vi "Initialize Lockin.vi"(8 "error in (no error)":errorcluster, 11 "Hardware Parameters":T1={"Scan Calibration [G/V]"=0.0, "Modulation Calibration [G/V]"=0.0, "Modulation Phase [deg]"=0.0, "Modulation Frequency [Hz]"=0.0, "Attenuation [dB]"=0, "Input Channel Count"=0, "Time constant"=7, "Sensitivity"=17, "Frequency Output Voltage [V]"=0.0, "Phase Output Voltage [V]"=0.0, "Lock-in Offset Compensation"=FALSE, "RF [GHz]"=0.0, "Q Start"=0.0, "Q End"=0.0, "Balance"=0.0, "Phase Error"=0.0, "AFC Error"=0.0, "AFC"=FALSE, "Magnet Rotation"=FALSE, "Balance Scaling Factor"=1.0, "Phase Error Scaling Factor"=1.0, "AFC Error Scaling Factor"=1.0, "Frequency Counter ID"="", "Sweep Waveform"=enum."Sawtooth", "Q-Factor Scale"=0.0, " Q-Data Scale"=0.0, " Q-Data Offset"=0.0, "Magnet Rotation Slope"=0.0, "Magnet Rotation Offset"=0.0, "Phase Sweep Resolution"=0.0, "Hardware Version Number"="", "Spectrometer ID Number"=0, "Spectrometer Name"="", "Lock in Saturation"=0.0, "Balance Threshold"=0.0, "Phase Error Threshold"=0.0, "AFC Error Threshold"=0.0, "Linear Actuator Length"=0.0, "Lock-in OK?"=FALSE, "Ignore Lock-in Comm. Failure"=FALSE, "Gradient Addresses"=[], "Gradient Calibrations [G/A*mm]"=[], "Gradient Power Supplies"=[], "Lock-in Address"="", "Magnet Type"=enum."RRI", "Camera Names"=[], "Sweep Limit [Gauss]"=0.0, "Modulation Limit [Gauss]"=0.0, "Balance Threshold Exceeded?"=FALSE, "Phase Threshold Exceeded?"=FALSE, "AFC Threshold Exceeded?"=FALSE, "Consecutive Re-tune attempts"=0, "Reverse Sweep Slope [sec]"=0.0, "Reverse Sweep Offset [G]"=0.0, "AFC Field Correction [V/MHz]"=0.0, "Active Gradients (X Y Z)"=[], "SpO2 Calibration [SpO2/V]"=1.0, "Heart Rate Calibration [BPM/V]"=1.0, "Thermocouple Channel"=""} {"Sensitivity" items=["", "2 nV", "5 nV", "10 nV", "20 nV", "50 nV", "100 nV", "200 nV", "500 nV", "1 uV", "2 uV", "5 uV", "10 uV", "20 uV", "50 uV", "100 uV", "200 uV", "500 uV", "1 mV", "2 mV", "5 mV", "10 mV", "20 mV", "50 mV", "100 mV", "200 mV", "500 mV", "1 V"]; "Time constant" items=["10 us", "20 us", "40 us", "80 us", "160 us", "320 us", "640 us", "5 ms", "10 ms", "20 ms", "50 ms", "100 ms", "200 ms", "500 ms", "1 s", "2 s", "5 s", "10 s", "20 s", "50 s", "100 s", "200 s", "500 s", "1 ks", "2 ks", "5 ks", "10 ks", "20 ks", "50 ks", "100 ks"]}) -> (0 "error out":errorcluster)   [LabVIEW 2016]
uses:
  Types/Hardware Parameters.ctl
panel:
  # "Bridge I/O"
  # "Magnet Rotation"
  # "Field Calibration"
  # "Lock In Amplifier"
  # "Spectrometer Information"
  # "DAQ Settings"
  # "Gradient Coils and Field"
  # "X"
  # "Y"
  # "Z"
  # "Q-Measurements"
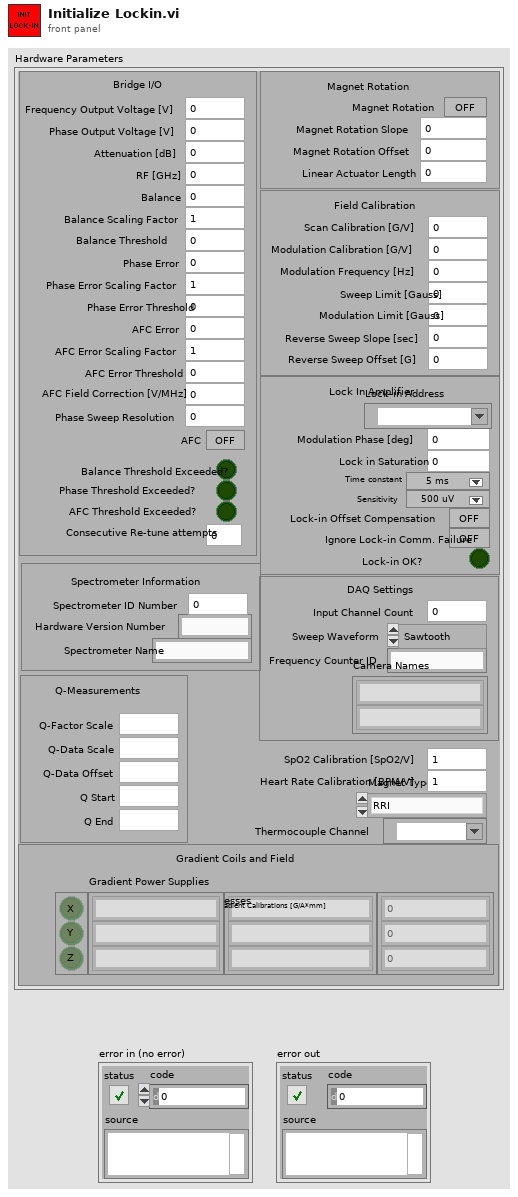
[diagram p1: front panel]
types:
  T1 = typedef "Hardware Parameters.ctl" = cluster{"Scan Calibration [G/V]":dbl, "Modulation Calibration [G/V]":dbl, "Modulation Phase [deg]":dbl, "Modulation Frequency [Hz]":dbl, "Attenuation [dB]":u16, "Input Channel Count":i32, "Time constant":u16, "Sensitivity":u16, "Frequency Output Voltage [V]":dbl, "Phase Output Voltage [V]":dbl, "Lock-in Offset Compensation":bool, "RF [GHz]":dbl, "Q Start":dbl, "Q End":dbl, "Balance":dbl, "Phase Error":dbl, "AFC Error":dbl, "AFC":bool, "Magnet Rotation":bool, "Balance Scaling Factor":dbl, "Phase Error Scaling Factor":dbl, "AFC Error Scaling Factor":dbl, "Frequency Counter ID":string, "Sweep Waveform":enum16{"Sine Wave", "Square Wave", "Sawtooth", "Triangle Wave"}, "Q-Factor Scale":dbl, " Q-Data Scale":dbl, " Q-Data Offset":dbl, "Magnet Rotation Slope":dbl, "Magnet Rotation Offset":dbl, "Phase Sweep Resolution":dbl, "Hardware Version Number":string, "Spectrometer ID Number":i32, "Spectrometer Name":string, "Lock in Saturation":dbl, "Balance Threshold":dbl, "Phase Error Threshold":dbl, "AFC Error Threshold":dbl, "Linear Actuator Length":dbl, "Lock-in OK?":bool, "Ignore Lock-in Comm. Failure":bool, "Gradient Addresses":string[], "Gradient Calibrations [G/A*mm]":dbl[], "Gradient Power Supplies":string[], "Lock-in Address":refnum<visa-resource-name>, "Magnet Type":enum16{"RRI", "BARDA", "Whole Body Permanent", "RRI Electromagnet"}, "Camera Names":string[], "Sweep Limit [Gauss]":dbl, "Modulation Limit [Gauss]":dbl, "Balance Threshold Exceeded?":bool, "Phase Threshold Exceeded?":bool, "AFC Threshold Exceeded?":bool, "Consecutive Re-tune attempts":i32, "Reverse Sweep Slope [sec]":dbl, "Reverse Sweep Offset [G]":dbl, "AFC Field Correction [V/MHz]":dbl, "Active Gradients (X Y Z)":bool[], "SpO2 Calibration [SpO2/V]":dbl, "Heart Rate Calibration [BPM/V]":dbl, "Thermocouple Channel":tag}
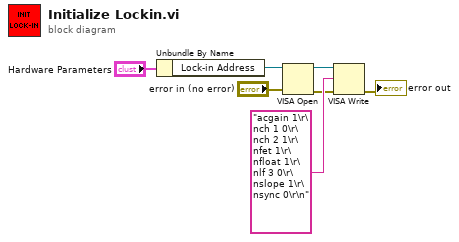
[diagram p0: block diagram]
diagram:
  n1 = Unbundle By Name("Hardware Parameters") -> ("Lock-in Address"=w1:refnum<visa-resource-name>)
  n2 = VISA Open(error in (no error)="error in (no error)", VISA resource name=w1) -> (VISA resource name=w6:refnum<visa-resource-name>, error out=w4:errorcluster)  [unwired: 3 out]
  n3 = VISA Write(VISA resource name=w6, write buffer="acgain 1\r\nch 1 0\r\nch 2 1\r\nfet 1\r\nfloat 1\r\nlf 3 0\r\nslope 1\r\nsync 0\r\n", error in (no error)=w4) -> (error out=→"error out":errorcluster)  [unwired: 2 out]
